vi "Current Loop 9505 (FPGA) - aft CombSampCurrLoop_bef CombPWMGenLoop.vi"() -> ()   [LabVIEW 2011]
uses:
  <vilib>/LabVIEW Targets/FPGA/cRIO/cRIO-9505/controls.llb/_nicrio_cRIO-9505_DriveStatus.ctl
  <vilib>/Platform/TimedLoop/XDataNode/timing_clust.ctl
  <vilib>/Platform/TimedLoop/XDataNode/nitl_modes.ctl
  <vilib>/Platform/TimedLoop/XDataNode/wakeup.ctl
  <vilib>/LabVIEW Targets/FPGA/cRIO/cRIO-9505/controls.llb/_nicrio_cRIO-9505_DriveDirection.ctl
  <vilib>/rvi/eio/common/nirviEmuTemplateMethod_errors.vi
  <vilib>/rvi/eio/common/nirviEmuTemplatePropertyGet_noerrors.vi
  <vilib>/Platform/TimedLoop/XDataNode/XDataNode.xnode
  <vilib>/eio/EIOMethodNode/EIOMethodNode.xnode
  <vilib>/eio/EIOPropertyNode/EIOPropertyNode.xnode
  <vilib>/eio/EIONode/EIONode.xnode
  <vilib>/Platform/TimedLoop/XDataNode/XDNodeRunTimeDep.lvlib
  <vilib>/rvi/eio/common/nirviEmuTemplatePropertyGet_errors.vi
  <vilib>/rvi/eio/common/nirviEmuTemplatePropertySet_errors.vi
  <vilib>/rvi/eio/common/nirviEmuTemplatePropertySet_noerrors.vi
panel:
  in  "Trig AI 2":bool
  out "Vsup Present 2":bool
  out "Drive Fault 2":bool
  out "Drive Status 2":T1
  out "Temp Fault 2":bool
  in  "Enable\nDrive 2":bool
  in  "Disable\nDrive 2":bool
  in  "Current PI gains 2":T2={"Proportional Gain"=20, "Integral Gain"=10, "Derivative Gain"=0}
  in  "Current Feedback 2":i16
  in  "Current Limit 2":i16 caption="Setpoint"
  in  "Current Setpoint 2":i16 caption="Setpoint"
  in  "Current Loop\nRate (usec) 2":u32=50
  out "PWM Duty Cycle 2":i16
  in  "Current PI gains":T2={"Proportional Gain"=20, "Integral Gain"=10, "Derivative Gain"=0}
  in  "Current Limit":i16 caption="Setpoint"
  in  "Current Setpoint":i16 caption="Setpoint"
  in  "Current Loop\nRate (usec)":u32=50
  out "Vsup Present":bool
  out "Drive Fault":bool
  out "Drive Status":T1
  out "Temp Fault":bool
  in  "Enable\nDrive":bool
  in  "Disable\nDrive":bool
  in  "Trig AI":bool
  in  "Current Feedback":i16
  out "PWM Duty Cycle":i16
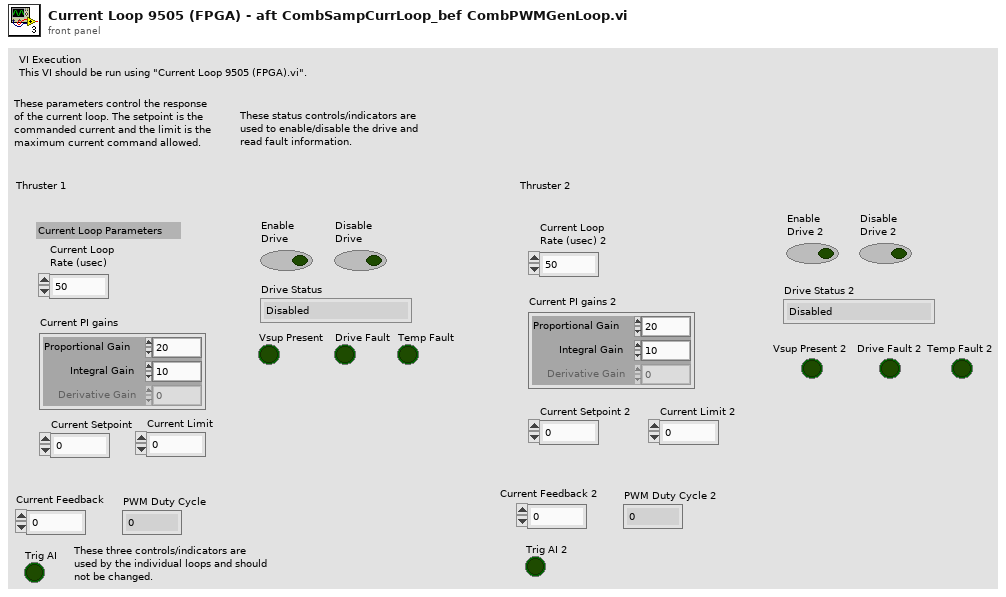
[diagram p1: front panel]
types:
  T1 = typedef "_nicrio_cRIO-9505_DriveStatus.ctl" = enum8{"Enabled", "Disabled", "Disabled by Drive Fault", "Disabled by Temp. Fault", "Disabled by E-Stop", "Unknown"}
  T2 = cluster{"Proportional Gain":i16, "Integral Gain":i16, "Derivative Gain":i16}
  T3 = typedef "XDNodeRunTimeDep.lvlib/timing_clust.ctl" = cluster{"Expected End [f-1]":u64, "Actual End [f-1]":u64, "Finished Late? [f-1]":bool, "Expected End [i-1]":u64, "Actual End [i-1]":u64, "Finished Late? [i-1]":bool, "Expected Start [i]":u64, "Actual Start [i]":u64, "Expected Start [f]":u64, "Actual Start [f]":u64, "Source Name":string, "Structure Name":string, "Period":i64, "Deadline":i64, "Offset":i64, "Start":i64, "Priority":i32, "Timeout":i32, "Mode":T4, "Wakeup Reason":T5, "Error":errorcluster, "Source Type":string, "Secondary Source Type":string, "Global End Time":u64, "Global Start Time":u64, "Frame Duration":u64, "Iteration Duration":u64, "Assigned CPU":i32, "I/O Scan Engine Mode":u32}
  T4 = typedef "XDNodeRunTimeDep.lvlib/nitl_modes.ctl" = enum32{"No Change", "Process missed periods, maintain original phase", "Discard missed periods, maintain original phase", "Process missed periods, ignore original phase", "Discard missed periods, ignore original phase"}
  T5 = typedef "XDNodeRunTimeDep.lvlib/wakeup.ctl" = enum32{"Normal", "Aborted", "Asynchronous wakeup", "Timing source error", "Timed loop error", "Timeout"}
  T6 = typedef "_nicrio_cRIO-9505_DriveDirection.ctl" = enum8{"Clockwise", "Counterclockwise"}
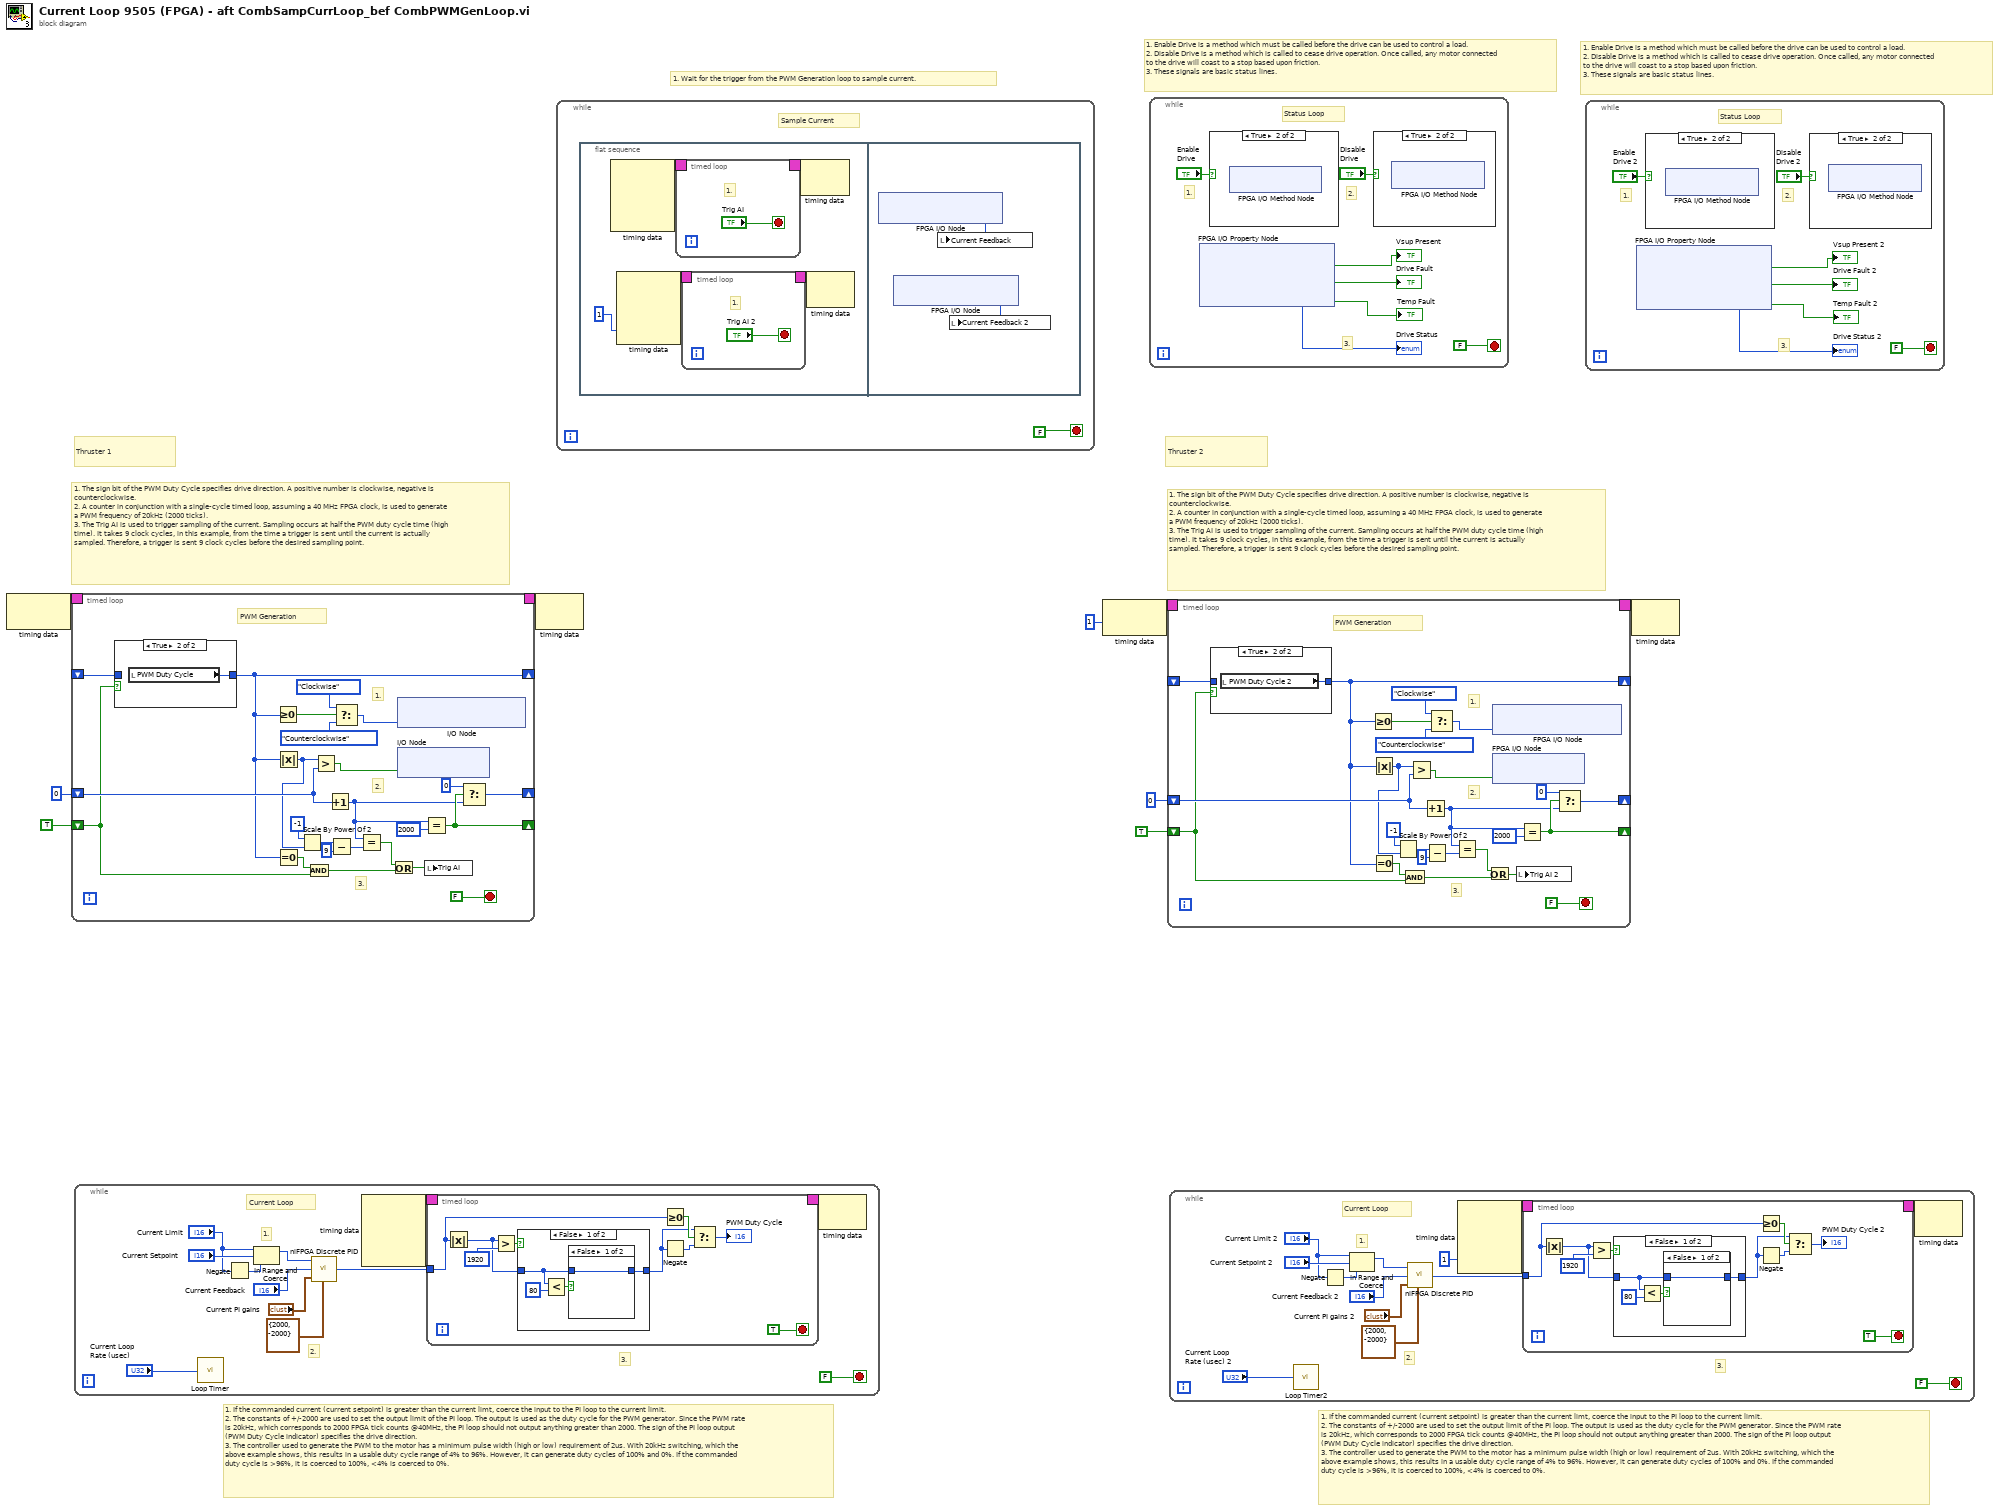
[diagram p0: block diagram]
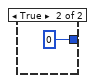
[diagram p5: hidden frame]
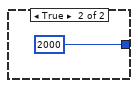
[diagram p6: hidden frame]
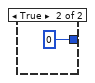
[diagram p10: hidden frame]
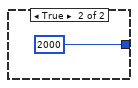
[diagram p11: hidden frame]
diagram:
  # "Thruster 2"
  # "Thruster 1"
  # "1. Enable Drive is a method which must be called before the drive can be used to control a load.\n2. Disable Drive is a method which is called to cease drive operation. Once called, any motor connected to the drive will coast to a stop based upon friction.\n3. These signals are basic status lines."
  # "1. Wait for the trigger from the PWM Generation loop to sample current."
  # "1. The sign bit of the PWM Duty Cycle specifies drive direction. A positive number is clockwise, negative is counterclockwise.\n2. A counter in conjunction with a single-cycle timed loop, assuming a 40 MHz FPGA clock, is used to generate a PWM frequency of 20kHz (2000 ticks).\n3. The Trig AI is used to trigger sampling of the current. Sampling occurs at half the PWM duty cycle time (high time). It takes 9 clock cycles, in this example, from the time a trigger is sent until the current is actually sampled. Therefore, a trigger is sent 9 clock cycles before the desired sampling point."
  # "1. If the commanded current (current setpoint) is greater than the current limt, coerce the input to the PI loop to the current limit.\n2. The constants of +/-2000 are used to set the output limit of the PI loop. The output is used as the duty cycle for the PWM generator. Since the PWM rate is 20kHz, which corresponds to 2000 FPGA tick counts @40MHz, the PI loop should not output anything greater than 2000. The sign of the PI loop output (PWM Duty Cycle indicator) specifies the drive direction.\n3. The controller used to generate the PWM to the motor has a minimum pulse width (high or low) requirement of 2us. With 20kHz switching, which the above example shows, this results in a usable duty cycle range of 4% to 96%. However, it can generate duty cycles of 100% and 0%. If the commanded duty c..."
  # "1. Enable Drive is a method which must be called before the drive can be used to control a load.\n2. Disable Drive is a method which is called to cease drive operation. Once called, any motor connected to the drive will coast to a stop based upon friction.\n3. These signals are basic status lines."
  # "1. The sign bit of the PWM Duty Cycle specifies drive direction. A positive number is clockwise, negative is counterclockwise.\n2. A counter in conjunction with a single-cycle timed loop, assuming a 40 MHz FPGA clock, is used to generate a PWM frequency of 20kHz (2000 ticks).\n3. The Trig AI is used to trigger sampling of the current. Sampling occurs at half the PWM duty cycle time (high time). It takes 9 clock cycles, in this example, from the time a trigger is sent until the current is actually sampled. Therefore, a trigger is sent 9 clock cycles before the desired sampling point."
  # "1. If the commanded current (current setpoint) is greater than the current limt, coerce the input to the PI loop to the current limit.\n2. The constants of +/-2000 are used to set the output limit of the PI loop. The output is used as the duty cycle for the PWM generator. Since the PWM rate is 20kHz, which corresponds to 2000 FPGA tick counts @40MHz, the PI loop should not output anything greater than 2000. The sign of the PI loop output (PWM Duty Cycle indicator) specifies the drive direction.\n3. The controller used to generate the PWM to the motor has a minimum pulse width (high or low) requirement of 2us. With 20kHz switching, which the above example shows, this results in a usable duty cycle range of 4% to 96%. However, it can generate duty cycles of 100% and 0%. If the commanded duty c..."
  n1 = node-c288() -> (w9:T3)  [unwired: 1 out]
  n2 = timed-loop {
    timing: w9 -> [_]
    timing-out: [_] -> w8
    shift-right: [w30] -> _
    shift-left: i16 0 -> [w33]
    shift-right: [w29] -> _
    shift-left: TRUE -> [w26]
    shift-right: [w15] -> _
    shift-left: _ -> [w28]
    stop <- FALSE stop-if-true
    # "3."
    # "2."
    # "1."
    # "PWM Generation"
    n3 = case shown="True" w26 {
      tunnel: [w34 w35] -> w15
      tunnel: w28 -> [w34 _]
      frame False {
      }
      frame True {
        n4 = local read "PWM Duty Cycle"() -> (w35:i16)
      }
    }
    n5 = Greater Or Equal To 0?(x=w15) -> (x >= 0?=w22:bool)
    n6 = Absolute Value(x=w15) -> (abs(x)=w13:i16)
    n7 = Equal To 0?(x=w15) -> (x = 0?=w27:bool)
    n8 = Scale By Power Of 2(n=i8 -1, x=w13) -> (x*2^n=w17:i16)
    n9 = And(x=w27, y=w26) -> (x .and. y?=w23:bool)
    n10 = Greater?(x=w13, y=w33) -> (0:w11:bool)
    n11 = Increment(x=w33) -> (x+1=w25:i16)
    n12 = Subtract(x=w17, y=i8 9) -> (x-y=w16:i16)
    n13 = Select(t=_nicrio_cRIO-9505_DriveDirection."Clockwise", s=w22, f=_nicrio_cRIO-9505_DriveDirection."Counterclockwise") -> (s? t:f=w10:T6)
    n14 = Equal?(x=w25, y=w16) -> (x = y?=w24:bool)
    n15 = Or(x=w24, y=w23) -> (x .or. y?=w19:bool)
    n16 = xnode "I/O Node"("Mod2/Drive Direction"=w10) -> ()  [unwired: 1 in, 1 out]
    n17 = xnode "I/O Node"("Mod2/Motor"=w11) -> ()  [unwired: 1 in, 1 out]
    n18 = Equal?(x=w25, y=i16 2000) -> (x = y?=w29:bool)
    n19 = local write "Trig AI"(w19) -> ()
    n20 = Select(t=i16 0, s=w29, f=w25) -> (s? t:f=w30:i16)
  }
  n21 = while {
    stop <- FALSE stop-if-true
    # "3."
    # "2."
    # "1."
    # "Current Loop"
    n22 = call "Loop Timer"("Count(uSec)"="Current Loop\nRate (usec)") -> ()  [unwired: 1 out]
    n23 = Negate(x="Current Limit") -> (-x=w42:i16)
    n24 = In Range and Coerce(upper limit="Current Limit", x="Current Setpoint", lower limit=w42) -> (coerced(x)=w40:i16)  [unwired: 1 out]
    n25 = call <vilib>:"niFPGA Discrete PID.vi"("setpoint"=w40, "process variable"="Current Feedback", "PID gains (x 2^8)"="Current PI gains", "output range"=cluster{"output high":i16, "output low":i16} {"output high"=2000, "output low"=-2000}) -> ("output"=w46:i16)  [unwired: 1 in, 4 out]
    n26 = node-c288() -> (w45:T3)  [unwired: 4 out]
    n27 = timed-loop {
      timing: w45 -> [_]
      timing-out: [_] -> w44
      tunnel: w46 -> [w52]
      stop <- TRUE stop-if-true
      n28 = Absolute Value(x=w52) -> (abs(x)=w53:i16)
      n29 = Greater?(x=w53, y=i16 1920) -> (0:w55:bool)
      n30 = case shown="False" w55 {
        tunnel: [w61 i16 2000] -> w54
        tunnel: w53 -> [w59 _]
        frame False {
          n31 = Less?(x=w59, y=i16 80) -> (x < y?=w60:bool)
          n32 = case shown="False" w60 {
            tunnel: [w63 i16 0] -> w61
            tunnel: w59 -> [w63 _]
            frame False {
            }
            frame True {
            }
          }
        }
        frame True {
        }
      }
      n33 = Greater Or Equal To 0?(x=w52) -> (x >= 0?=w58:bool)
      n34 = Negate(x=w54) -> (-x=w57:i16)
      n35 = Select(t=w54, s=w58, f=w57) -> (s? t:f=→"PWM Duty Cycle":i16)
    }
    n36 = node-c288(w44) -> ()  [unwired: 1 out]
  }
  n37 = node-c288(w8) -> ()  [unwired: 1 out]
  n38 = while {
    stop <- FALSE stop-if-true
    # "Sample Current"
    n39 = flat-sequence {
      frame #0 {
        n40 = node-c288() -> (w75:T3)  [unwired: 4 out]
        n41 = node-c288(1) -> (w73:T3)  [unwired: 3 out]
        n42 = timed-loop {
          timing: w75 -> [_]
          timing-out: [_] -> w74
          stop <- "Trig AI" stop-if-true
          # "1."
        }
        n43 = timed-loop {
          timing: w73 -> [_]
          timing-out: [_] -> w72
          stop <- "Trig AI 2" stop-if-true
          # "1."
        }
        n44 = node-c288(w74) -> ()  [unwired: 1 out]
        n45 = node-c288(w72) -> ()  [unwired: 1 out]
      }
      frame #1 {
        n46 = xnode "FPGA I/O Node"() -> ("Mod2/Current Sense"=w89:i16)  [unwired: 1 in, 1 out]
        n47 = xnode "FPGA I/O Node"() -> ("Mod4/Current Sense"=w88:i16)  [unwired: 1 in, 1 out]
        n48 = local write "Current Feedback"(w89) -> ()
        n49 = local write "Current Feedback 2"(w88) -> ()
      }
    }
  }
  n50 = node-c288(1) -> (w5:T3)
  n51 = while {
    stop <- FALSE stop-if-true
    # "3."
    # "2."
    # "1."
    # "Status Loop"
    n52 = xnode "FPGA I/O Property Node"() -> ("Vsup Present"=→"Vsup Present":bool, "Drive Fault"=→"Drive Fault":bool, "Drive Status"=→"Drive Status":T1, "Over Temperature Fault"=→"Temp Fault":bool)  [unwired: 1 in, 1 out]
    n53 = case shown="True" "Enable\nDrive" {
      frame False {
      }
      frame True {
        n54 = xnode "FPGA I/O Method Node"() -> ()  [unwired: 1 in, 1 out]
      }
    }
    n55 = case shown="True" "Disable\nDrive" {
      frame False {
      }
      frame True {
        n56 = xnode "FPGA I/O Method Node"() -> ()  [unwired: 1 in, 1 out]
      }
    }
  }
  n57 = timed-loop {
    timing: w5 -> [_]
    timing-out: [_] -> w4
    shift-right: [w117] -> _
    shift-left: i16 0 -> [w120]
    shift-right: [w116] -> _
    shift-left: TRUE -> [w113]
    shift-right: [w102] -> _
    shift-left: _ -> [w115]
    stop <- FALSE stop-if-true
    # "3."
    # "2."
    # "1."
    # "PWM Generation"
    n58 = case shown="True" w113 {
      tunnel: [w121 w122] -> w102
      tunnel: w115 -> [w121 _]
      frame False {
      }
      frame True {
        n59 = local read "PWM Duty Cycle 2"() -> (w122:i16)
      }
    }
    n60 = Greater Or Equal To 0?(x=w102) -> (x >= 0?=w109:bool)
    n61 = Absolute Value(x=w102) -> (abs(x)=w100:i16)
    n62 = Equal To 0?(x=w102) -> (x = 0?=w114:bool)
    n63 = Scale By Power Of 2(n=i8 -1, x=w100) -> (x*2^n=w104:i16)
    n64 = And(x=w114, y=w113) -> (x .and. y?=w110:bool)
    n65 = Greater?(x=w100, y=w120) -> (0:w98:bool)
    n66 = Increment(x=w120) -> (x+1=w112:i16)
    n67 = Subtract(x=w104, y=i8 9) -> (x-y=w103:i16)
    n68 = Select(t=_nicrio_cRIO-9505_DriveDirection."Clockwise", s=w109, f=_nicrio_cRIO-9505_DriveDirection."Counterclockwise") -> (s? t:f=w97:T6)
    n69 = Equal?(x=w112, y=w103) -> (x = y?=w111:bool)
    n70 = Or(x=w111, y=w110) -> (x .or. y?=w106:bool)
    n71 = xnode "FPGA I/O Node"("Mod4/Drive Direction"=w97) -> ()  [unwired: 1 in, 1 out]
    n72 = xnode "FPGA I/O Node"("Mod4/Motor"=w98) -> ()  [unwired: 1 in, 1 out]
    n73 = local write "Trig AI 2"(w106) -> ()
    n74 = Equal?(x=w112, y=i16 2000) -> (x = y?=w116:bool)
    n75 = Select(t=i16 0, s=w116, f=w112) -> (s? t:f=w117:i16)
  }
  n76 = while {
    stop <- FALSE stop-if-true
    # "3."
    # "2."
    # "1."
    # "Current Loop"
    n77 = call "Loop Timer2"("Count(uSec)"="Current Loop\nRate (usec) 2") -> ()  [unwired: 1 out]
    n78 = Negate(x="Current Limit 2") -> (-x=w130:i16)
    n79 = In Range and Coerce(upper limit="Current Limit 2", x="Current Setpoint 2", lower limit=w130) -> (coerced(x)=w128:i16)  [unwired: 1 out]
    n80 = call <vilib>:"niFPGA Discrete PID.vi"("setpoint"=w128, "process variable"="Current Feedback 2", "PID gains (x 2^8)"="Current PI gains 2", "output range"=cluster{"output high":i16, "output low":i16} {"output high"=2000, "output low"=-2000}) -> ("output"=w134:i16)  [unwired: 1 in, 4 out]
    n81 = node-c288(1) -> (w133:T3)  [unwired: 3 out]
    n82 = timed-loop {
      timing: w133 -> [_]
      timing-out: [_] -> w132
      tunnel: w134 -> [w140]
      stop <- TRUE stop-if-true
      n83 = Absolute Value(x=w140) -> (abs(x)=w141:i16)
      n84 = Greater?(x=w141, y=i16 1920) -> (0:w143:bool)
      n85 = case shown="False" w143 {
        tunnel: [w149 i16 2000] -> w142
        tunnel: w141 -> [w147 _]
        frame False {
          n86 = Less?(x=w147, y=i16 80) -> (x < y?=w148:bool)
          n87 = case shown="False" w148 {
            tunnel: [w151 i16 0] -> w149
            tunnel: w147 -> [w151 _]
            frame False {
            }
            frame True {
            }
          }
        }
        frame True {
        }
      }
      n88 = Greater Or Equal To 0?(x=w140) -> (x >= 0?=w146:bool)
      n89 = Negate(x=w142) -> (-x=w145:i16)
      n90 = Select(t=w142, s=w146, f=w145) -> (s? t:f=→"PWM Duty Cycle 2":i16)
    }
    n91 = node-c288(w132) -> ()  [unwired: 1 out]
  }
  n92 = while {
    stop <- FALSE stop-if-true
    # "3."
    # "2."
    # "1."
    # "Status Loop"
    n93 = xnode "FPGA I/O Property Node"() -> ("Vsup Present"=→"Vsup Present 2":bool, "Drive Fault"=→"Drive Fault 2":bool, "Drive Status"=→"Drive Status 2":T1, "Over Temperature Fault"=→"Temp Fault 2":bool)  [unwired: 1 in, 1 out]
    n94 = case shown="True" "Enable\nDrive 2" {
      frame False {
      }
      frame True {
        n95 = xnode "FPGA I/O Method Node"() -> ()  [unwired: 1 in, 1 out]
      }
    }
    n96 = case shown="True" "Disable\nDrive 2" {
      frame False {
      }
      frame True {
        n97 = xnode "FPGA I/O Method Node"() -> ()  [unwired: 1 in, 1 out]
      }
    }
  }
  n98 = node-c288(w4) -> ()  [unwired: 1 out]
